vi "Score.vi"(7 "Mov_Spd":i32, 8 "error in":errorcluster, 10 "Obs D_in":refnum<vi>[](array[refnum]), 11 "Ball in":refnum<vi>) -> (0 "error out":errorcluster, 2 "Msg":string, 3 "Add":i32)   [LabVIEW 8.6]
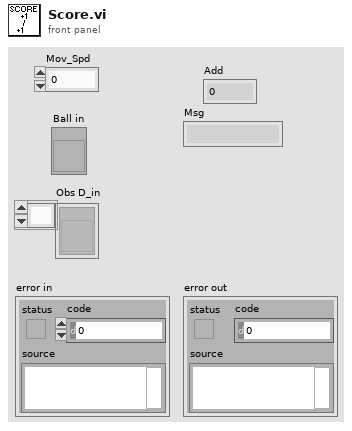
[diagram p1: front panel]
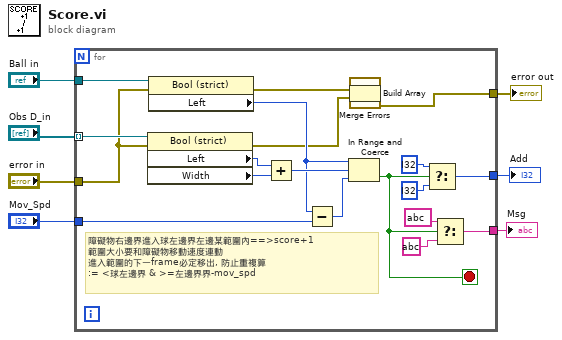
[diagram p0: block diagram]
diagram:
  n1 = for {
    tunnel: "Mov_Spd" -> [w27]
    tunnel: [w23] -> w6
    tunnel: "Ball in" -> [w16]
    tunnel: "Obs D_in" -> [w15] mode=indexing
    tunnel: [w14] -> w4
    tunnel: "error in" -> [w13]
    tunnel: [w11] -> w1
    stop <- w12 stop-if-true
    # "障礙物右邊界進入球左邊界左邊某範圍內==>score+1\n範圍大小要和障礙物移動速度連動\n進入範圍的下一frame必定移出, 防止重複算\n:= <球左邊界 & >=左邊界界-mov_spd"
    n2 = property on="Property Node" class="Bool (strict)"(reference=w15, error in=w13) -> (error out=w21:errorcluster, "Left"=w20:i32, "Width"=w19:u32)  [unwired: 1 out]
    n3 = property on="Property Node" class="Bool (strict)"(reference=w16, error in=w13) -> (error out=w22:errorcluster, "Left"=w24:i32)  [unwired: 1 out]
    n4 = Add(x=w20, y=w19) -> (x+y=w26:u32)
    n5 = Subtract(x=w24, y=w27) -> (x-y=w25:i32)
    n6 = In Range and Coerce(upper limit=w24, x=w26, lower limit=w25) -> (In Range?=w12:bool)  [unwired: 1 out]
    n7 = Build Array(w22, w21) -> (w8:errorcluster[])
    n8 = call <vilib>:"Merge Errors.vi"("error array in"=w8) -> ("error out"=w14:errorcluster)  [unwired: 6 in]
    n9 = Select(t=i32 ?, s=w12, f=i32 ? ("t")) -> (s? t:f=w23:i32)
    n10 = Select(t=string ?, s=w12, f=string ?) -> (s? t:f=w11:string)
  }
  "Add" <- w6
  "error out" <- w4
  "Msg" <- w1
